vi "Highlight State Call.vi"(8 "error in (no error)":errorcluster, 10 "Cluster":T1, 11 "JKI SM in":refnum<class "JKI SM.lvclass">) -> (0 "error out":errorcluster, 3 "JKI SM out":refnum<class "JKI SM.lvclass">)   [LabVIEW 2013]
uses:
  JKI State Machine API/source/JKI SM/JKI SM.lvclass
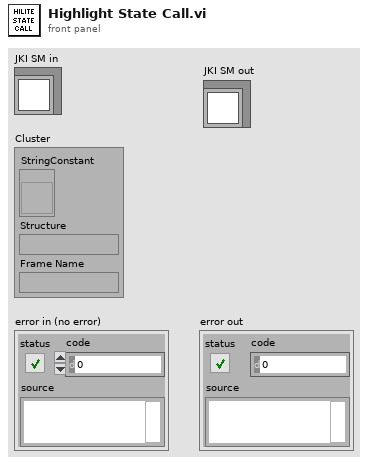
[diagram p1: front panel]
types:
  T1 = cluster{"StringConstant":refnum<vi>, "Structure":string, "Frame Name":string}
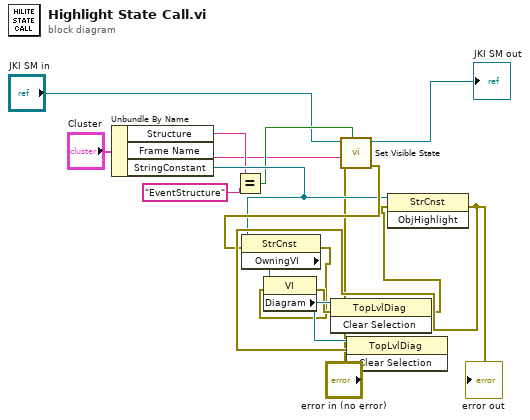
[diagram p0: block diagram]
diagram:
  n1 = Unbundle By Name("Cluster") -> ("Structure"=w7:string, "Frame Name"=w4:string, "StringConstant"=w9:refnum<vi>)
  n2 = Equal?(x=w7, y="EventStructure") -> (x = y?=w8:bool)
  n3 = call "Set Visible State.vi"("Event Structure (F: Case Structure)"=w8, "error in (no error)"="error in (no error)", "State Name"=w4, "JKI SM in"="JKI SM in") -> ("error out"=w11:errorcluster, "JKI SM out"=→"JKI SM out":refnum<class "JKI SM.lvclass">)  [unwired: 6 in]
  n4 = property class="StrCnst"(reference=w9, error in=w11) -> (error out=w12:errorcluster, "OwningVI"=w10:refnum<vi>)  [unwired: 1 out]
  n5 = property class="VI"(reference=w10, error in=w12) -> (error out=w13:errorcluster, "Diagram"=w16:refnum<vi>)  [unwired: 1 out]
  n6 = invoke class="TopLvlDiag" method="Clear Selection"(reference=w16, error in=w13) -> (error out=w14:errorcluster)  [unwired: 1 in, 2 out]
  n7 = invoke class="StrCnst" method="ObjHighlight"(reference=w9, error in=w14) -> (error out=w15:errorcluster)  [unwired: 1 in, 2 out]
  "error out" <- w15
  n8 = invoke class="TopLvlDiag" method="Clear Selection"(reference=w16, error in=w15) -> ()  [unwired: 1 in, 3 out]
